vi "PH_PPMA_PowerUnit.PS Switch PU on.vi"(0 "i ref in":refnum<vi>, 5 "error in (no error)":errorcluster) -> (14 "i ref out":refnum<vi>, 19 "error out":errorcluster)   [LabVIEW 2014, in "PH_PPMA_PowerUnit.lvlib"]
uses:
  PH_PPMA_PowerUnit.lvlib
  PH_Beckhoff_PPMA-Rods/PH_Beckhoff_PPMA-Rods.lvlib
  PH_Beckhoff_PP_PU/PH_Beckhoff_PP_PU.lvlib
  PH_PowerUnit_BaseClass/PH_PowerUnit_BaseClass.lvlib
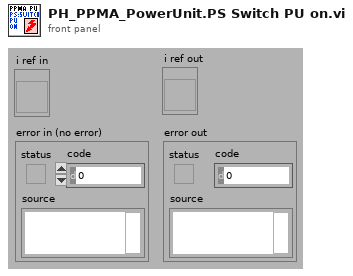
[diagram p1: front panel]
types:
  T1 = typedef "PH_PPMA_PowerUnit.lvlib/PH_PPMA_PowerUnit.i attribute.ctl" = cluster{"GUI Refs":cluster{"Rods":refnum<vi>, "Ignitron":refnum<vi>, "Rossrelais":refnum<vi>, "Set Voltage":refnum<vi>, "PSU":refnum<vi>, "EOC":refnum<vi>, "Trigger":refnum<vi>}, "Rods":T2, "PSU":T4, "Ross Relais":T5, "Ignitron":T6, "Trigger":cluster{"State Device":T3, "linked?":bool}, "Timing Settings":cluster{"Prdc Fast?":bool, "Default Value Periodic Interval":i32, "Mercury on since":dbl, "Warm up Time Mercury [s]":dbl}, "Set Voltage [V]":dbl}
  T2 = typedef "PH_PPMA_PowerUnit.lvlib/PH_PPMA_PowerUnit.Rods Attributes.ctl" = cluster{"Instancename":string, "Device Status":T3, "linked?":bool}
  T3 = typedef "PH_StatusHandler.lvlib/PH_StatusHandler.Status.ctl" = i16
  T4 = typedef "PH_PP_Common.lvlib/PH_PP_Common.PSU Attributes.ctl" = cluster{"lower limit [V]":dbl, "upper limit [V]":dbl, "Voltage set":bool, "State Device":T3, "linked?":bool}
  T5 = typedef "PH_PP_Common.lvlib/PH_PP_Common.Ross Relais Attributes.ctl" = cluster{"State Device":T3, "linked?":bool}
  T6 = typedef "PH_PP_Common.lvlib/PH_PP_Common.Ignitron Attributes.ctl" = cluster{"State Device":T3, "linked?":bool}
  T7 = typedef "PH_PowerUnit_BaseClass.lvlib/PH_PowerUnit_BaseClass.i attribute.ctl" = cluster{"Constructor finished":bool, "PU":cluster{"In use":bool, "Service ID in use":i32, "GUI Ref":refnum<vi>}, "Enabling":cluster{"State":T8, "GUI Ref":refnum<vi>}, "Timing":cluster{"Last Shot":dbl, "Time between Shots [Sec]":dbl, "Waiting Time over?":bool, "Service ID Waiting Time":i32, "GUI Ref":refnum<vi>, "Instance":cluster{"Status":T3, "linked?":bool, "GUI Ref":refnum<vi>}}, "Sequencer":cluster{"SM State":string, "GUI Ref":refnum<vi>, "linked":bool}, "Subscribed Trendmssgs":cluster{"Tagname":string, "Status":T3, "linked?":bool, "Shot Condition":T3, "GUI Ref":refnum<vi>}[], "PP PU":T9, "Default Voltage (V)":dbl, "GUI Refs":T10, "PSDB data":cluster{"Shot Voltage [V]":dbl, "State TO SM":T11, "Write 2 early":bool}, "State TO SM":T11}
  T8 = typedef "PH_SystemInformation.lvlib/PH_SystemInformationEnabling State.ctl" = i32
  T9 = typedef "PH_PP_Common.lvlib/PH_PP_Common.PUs.ctl" = enum16{"no Info", "PA-19mm-1", "PA-19mm-2", "PA-45mm-PILC", "PA-45mm-MAIN", "MA-PU-1", "MA-PU-2", "MA-PU-3", "MA-PU-4", "MA-PU-5", "MA-PU-6", "MA-FR", "MA-PILC", "PA-45mm-DP"}
  T10 = typedef "PH_PowerUnit_BaseClass.lvlib/PH_PowerUnit_BaseClass.GUI Refs.ctl" = cluster{"Delete Inst":refnum<vi>, "State TO SM":refnum<vi>, "State SM":refnum<vi>, "Fire":refnum<vi>}
  T11 = typedef "PH_PowerUnit_BaseClass.lvlib/PH_PowerUnit_BaseClass.SM States.ctl" = enum16{".", "Stand by", "Switch PU on", "Configure", "Set Default Voltage", "Set STANDBY", "Set READY", "Wait for Shot Cmd", "Open Dump Rods", "Open Ross Relais", "Close Ross Relais", "Switch PSU on", "Switch PSU off", "Charge", "Switch GD Channel on", "Close Dump Rods", "Rods-TO", "RR-TO", "PSU-TO", "Trigger-TO"}
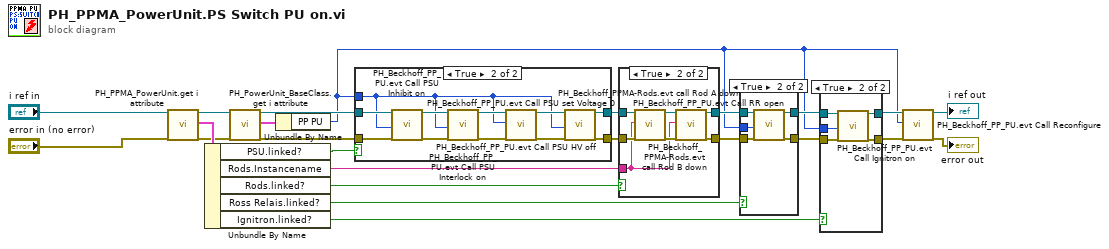
[diagram p0: block diagram]
diagram:
  n1 = call "PH_PPMA_PowerUnit.get i attribute.vi"("i ref in"="i ref in", "error in (no error)"="error in (no error)") -> ("i ref out"=w23:refnum<vi>, "i attribute"=w24:T1, "error out"=w6:errorcluster)  [unwired: 15 in]
  n2 = Unbundle By Name(w24) -> ("PSU.linked?"=w16:bool, "Rods.Instancename"=w15:string, "Rods.linked?"=w14:bool, "Ross Relais.linked?"=w13:bool, "Ignitron.linked?"=w12:bool)
  n3 = call "PH_PowerUnit_BaseClass.get i attribute.vi"("i ref in"=w23, "error in (no error)"=w6) -> ("i ref out"=w7:refnum<vi>, "i attribute"=w4:T7, "error out"=w5:errorcluster)  [unwired: 15 in]
  n4 = Unbundle By Name(w4) -> ("PP PU"=w1:T9)
  n5 = case shown="True" w16 {
    tunnel: w7 -> [w26 w37]
    tunnel: [w26 w33] -> w17
    tunnel: w5 -> [w25 w32]
    tunnel: [w25 w28] -> w20
    tunnel: w1 -> [_ w27]
    frame False {
    }
    frame True {
      n6 = call "PH_Beckhoff_PP_PU.evt Call PSU Inhibit on.vi"("i ref in"=w37, "PU"=w27, "error in"=w32) -> ("i ref out"=w36:refnum<vi>, "error out"=w31:errorcluster)  [unwired: 15 in]
      n7 = call "PH_Beckhoff_PP_PU.evt Call PSU Interlock on.vi"("i ref in"=w36, "PU"=w27, "error in"=w31) -> ("i ref out"=w35:refnum<vi>, "error out"=w30:errorcluster)  [unwired: 15 in]
      n8 = call "PH_Beckhoff_PP_PU.evt Call PSU set Voltage 0.vi"("i ref in"=w35, "PU"=w27, "error in"=w30) -> ("i ref out"=w34:refnum<vi>, "error out"=w29:errorcluster)  [unwired: 15 in]
      n9 = call "PH_Beckhoff_PP_PU.evt Call PSU HV off.vi"("i ref in"=w34, "PU"=w27, "error in"=w29) -> ("i ref out"=w33:refnum<vi>, "error out"=w28:errorcluster)  [unwired: 15 in]
    }
  }
  n10 = case shown="True" w14 {
    tunnel: w17 -> [w39 w46]
    tunnel: [w39 w41] -> w18
    tunnel: w20 -> [w38 w45]
    tunnel: [w38 w43] -> w21
    tunnel: w15 -> [_ w40]
    frame False {
    }
    frame True {
      n11 = call "PH_Beckhoff_PPMA-Rods.evt call Rod A down.vi"("i ref in"=w46, "Instance name"=w40, "error in"=w45) -> ("i ref out"=w42:refnum<vi>, "error out"=w44:errorcluster)  [unwired: 15 in]
      n12 = call "PH_Beckhoff_PPMA-Rods.evt call Rod B down.vi"("i ref in"=w42, "Instance name"=w40, "error in"=w44) -> ("i ref out"=w41:refnum<vi>, "error out"=w43:errorcluster)  [unwired: 15 in]
    }
  }
  n13 = case shown="True" w13 {
    tunnel: w18 -> [w48 w53]
    tunnel: [w48 w52] -> w19
    tunnel: w21 -> [w47 w51]
    tunnel: [w47 w50] -> w22
    tunnel: w1 -> [_ w49]
    frame False {
    }
    frame True {
      n14 = call "PH_Beckhoff_PP_PU.evt Call RR open.vi"("i ref in"=w53, "PU"=w49, "error in"=w51) -> ("i ref out"=w52:refnum<vi>, "error out"=w50:errorcluster)  [unwired: 15 in]
    }
  }
  n15 = case shown="True" w12 {
    tunnel: w19 -> [w55 w60]
    tunnel: [w55 w59] -> w8
    tunnel: w22 -> [w54 w58]
    tunnel: [w54 w57] -> w10
    tunnel: w1 -> [_ w56]
    frame False {
    }
    frame True {
      n16 = call "PH_Beckhoff_PP_PU.evt Call Ignitron on.vi"("i ref in"=w60, "PU"=w56, "error in"=w58) -> ("i ref out"=w59:refnum<vi>, "error out"=w57:errorcluster)  [unwired: 15 in]
    }
  }
  n17 = call "PH_Beckhoff_PP_PU.evt Call Reconfigure.vi"("i ref in"=w8, "Instance name"=w1, "error in"=w10) -> ("i ref out"=→"i ref out":refnum<vi>, "error out"=→"error out":errorcluster)  [unwired: 15 in]
